vi "堆物理参数设置.vi"() -> ()   [LabVIEW 2020]
uses:
  global/SettingVariable.vi
  <vilib>/Utility/config.llb/Write Key (Double).vi
  GlobalVariable.vi
  TCPModbus_MasterClient/MB Ethernet Master Query Write Multiple Registers (poly).vi
  <vilib>/Utility/config.llb/NI_LVConfig.lvlib
panel:
  in  "下发":bool
  in  "Lamda 6":sgl caption="Lamda 6:"
  in  "Lamda 5":sgl caption="Lamda 5:"
  in  "Lamda 4":sgl caption="Lamda 4:"
  in  "Lamda 3":sgl caption="Lamda 3:"
  in  "Lamda 2":sgl caption="Lamda 2:"
  in  "βeff 6":sgl caption="βeff 6:"
  in  "βeff 5":sgl caption="βeff 5:"
  in  "βeff 4":sgl caption="βeff 4:"
  in  "βeff 3":sgl caption="βeff 3:"
  in  "βeff 2":sgl caption="βeff 2:"
  in  "取消":bool caption="Cancel Button"
  in  "确定":bool
  in  "Lamda 1":sgl caption="Lamda 1:"
  in  "βeff 1":sgl caption="βeff 1:"
  in  "源强":sgl caption="源强(n/cm2·s):"
  in  "中子寿命":sgl caption="中子寿命(s):"
  # "中子学参数"
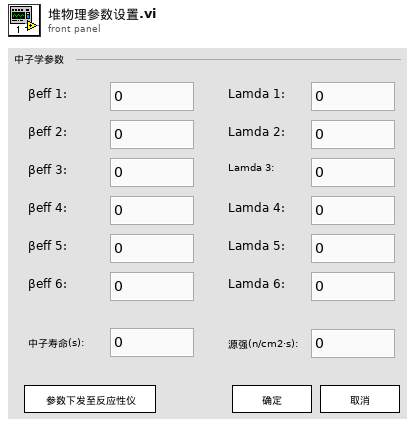
[diagram p1: front panel]
types:
  T1 = typedef "NI_LVConfig.lvlib/Config Data RefNum.ctl" = refnum<k1>
  T2 = enum32{"Bad", "Idle", "Run top level", "Running"}
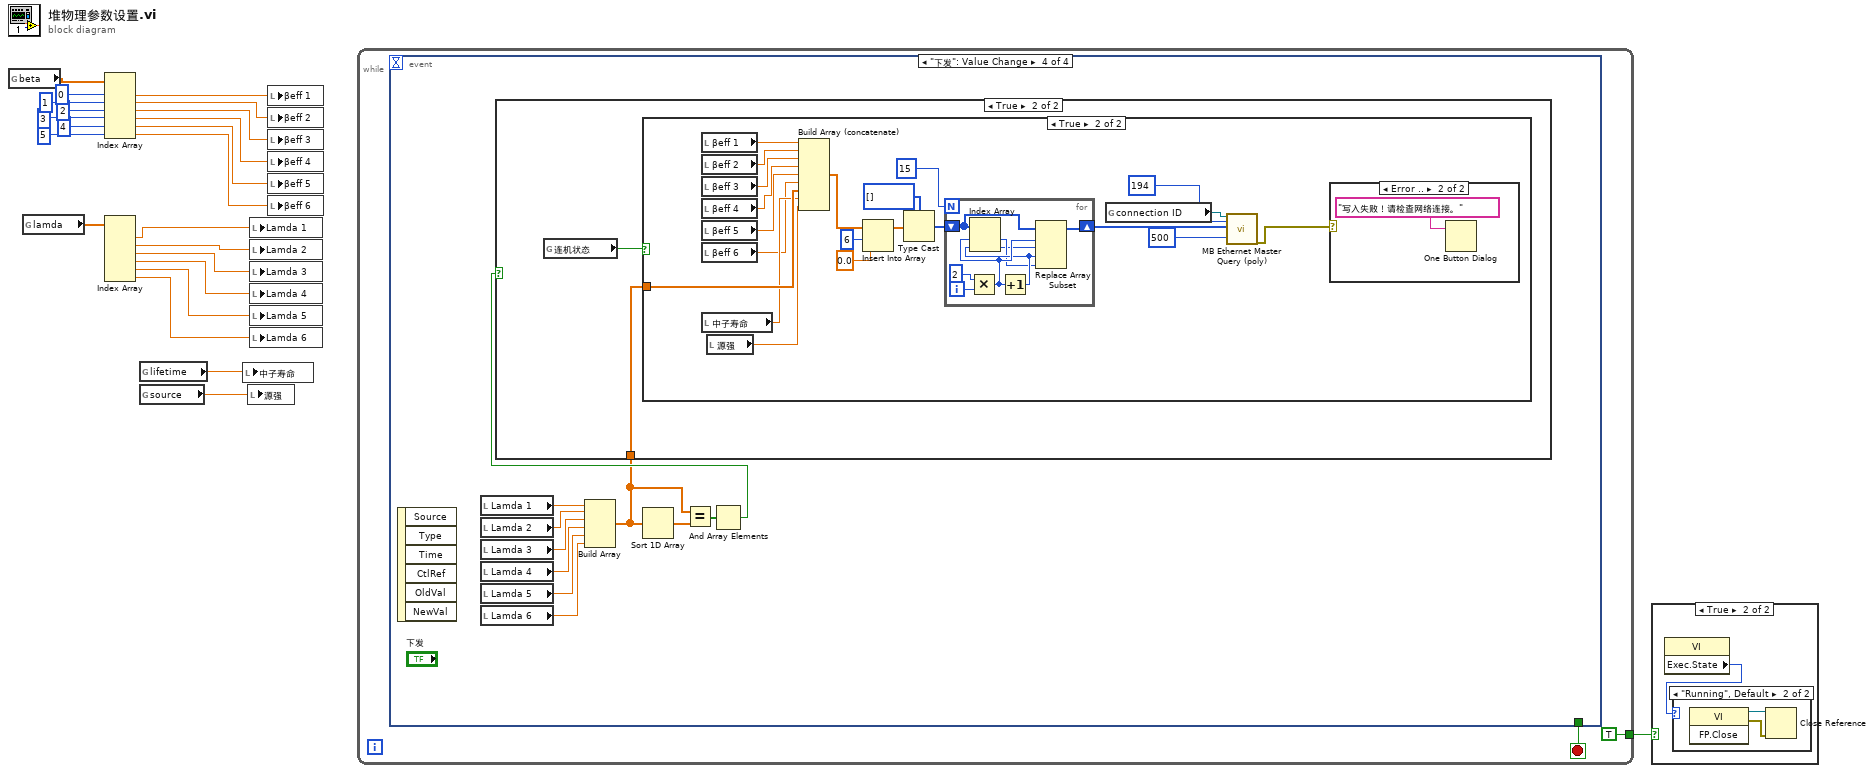
[diagram p0: block diagram]
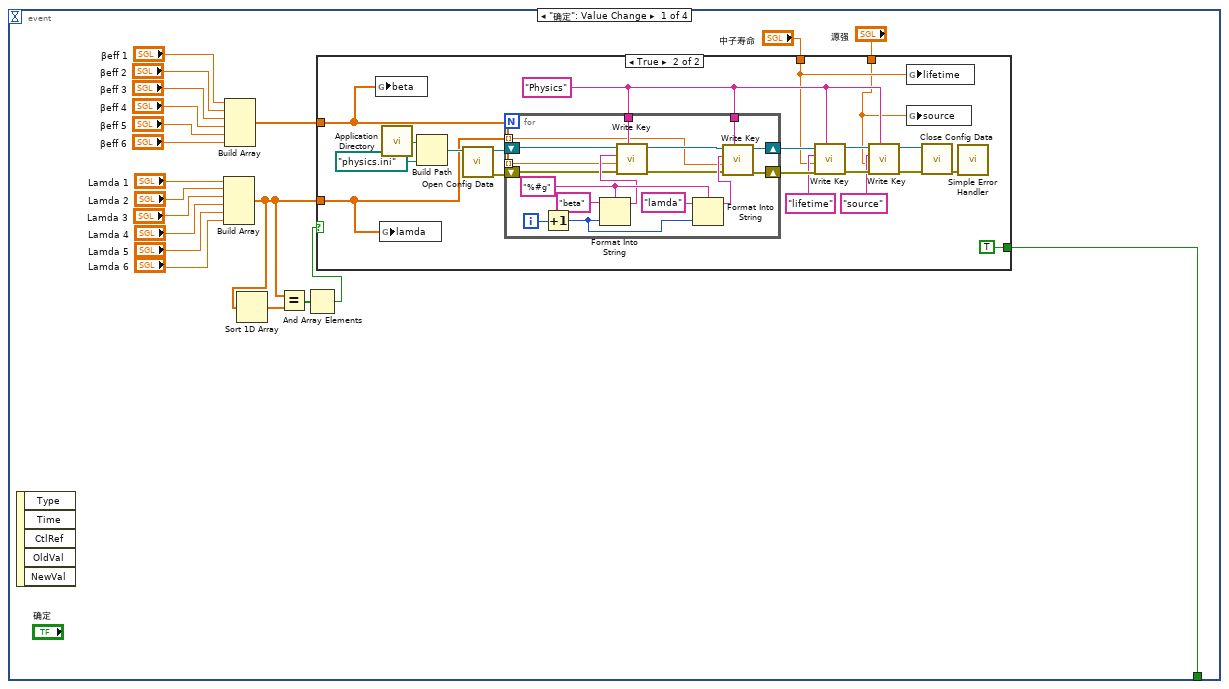
[diagram p4: hidden frame]
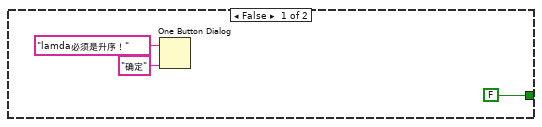
[diagram p5: hidden frame]
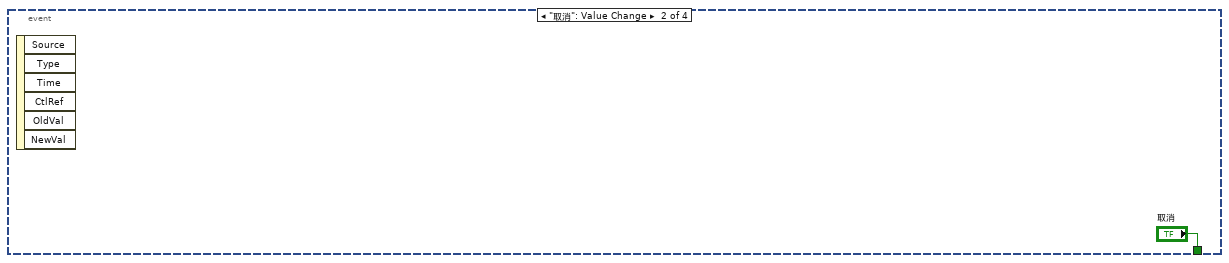
[diagram p6: hidden frame]
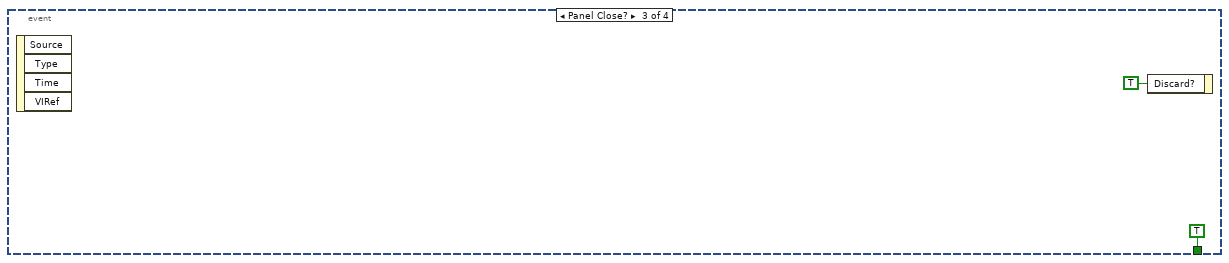
[diagram p7: hidden frame]
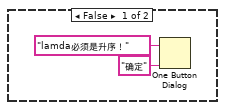
[diagram p8: hidden frame]
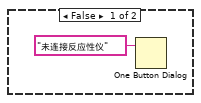
[diagram p9: hidden frame]
diagram:
  n1 = global read "SettingVariable.vi" "beta"() -> (w9:dbl[])
  n2 = global read "SettingVariable.vi" "lamda"() -> (w10:dbl[])
  n3 = Index Array(array=w9, index #1=0, index #2=1, index #3=2, index #4=3, index #5=4, index #6=5) -> (element #1=w17:dbl, element #2=w16:dbl, element #3=w15:dbl, element #4=w14:dbl, element #5=w13:dbl, element #6=w12:dbl)
  n4 = Index Array(array=w10) -> (element #1=w3:dbl, element #2=w4:dbl, element #3=w5:dbl, element #4=w6:dbl, element #5=w7:dbl, element #6=w8:dbl)  [unwired: 6 in]
  n5 = global read "SettingVariable.vi" "lifetime"() -> (w2:dbl)
  n6 = global read "SettingVariable.vi" "source"() -> (w1:dbl)
  n7 = local write "中子寿命"(w2) -> ()
  n8 = local write "源强"(w1) -> ()
  n9 = local write "Lamda 1"(w3) -> ()
  n10 = local write "Lamda 2"(w4) -> ()
  n11 = local write "Lamda 3"(w5) -> ()
  n12 = local write "Lamda 4"(w6) -> ()
  n13 = local write "Lamda 5"(w7) -> ()
  n14 = local write "Lamda 6"(w8) -> ()
  n15 = local write "βeff 1"(w17) -> ()
  n16 = local write "βeff 2"(w16) -> ()
  n17 = local write "βeff 3"(w15) -> ()
  n18 = local write "βeff 4"(w14) -> ()
  n19 = local write "βeff 5"(w13) -> ()
  n20 = local write "βeff 6"(w12) -> ()
  n21 = while {
    tunnel: [TRUE ("确定")] -> w11
    stop <- w25 stop-if-true
    n22 = event shown="[3] \"下发\": Value Change" {
      selector: _ -> [_ _ _ _]
      dyn-events: _ -> [_ _ _ _]
      timeout: _ -> [_ _ _ _]
      tunnel: [w26 "取消" TRUE ("确定") _] -> w25
      event "确定": Value Change {
        n23 = event-data() -> ()  [unwired: 1 in, 5 out]
        n24 = Build Array("Lamda 1", "Lamda 2", "Lamda 3", "Lamda 4", "Lamda 5", "Lamda 6") -> (w30:sgl[])
        n25 = Build Array("βeff 1", "βeff 2", "βeff 3", "βeff 4", "βeff 5", "βeff 6") -> (w33:sgl[])
        n26 = Sort 1D Array(array=w30) -> (sorted array=w29:sgl[])
        n27 = Equal?(x=w30, y=w29) -> (x = y?=w28:bool[])
        n28 = And Array Elements(Boolean array=w28) -> (logical AND=w27:bool)
        n29 = case shown="True" w27 {
          tunnel: w33 -> [_ w52]
          tunnel: w30 -> [_ w53]
          tunnel: "中子寿命" -> [_ w51]
          tunnel: "源强" -> [_ w50]
          tunnel: [FALSE ("确定") TRUE ("确定")] -> w26
          frame False {
            n30 = One Button Dialog(message="lamda必须是升序！", button name ("OK")="确定") -> ()  [unwired: 1 out]
          }
          frame True {
            w62 = "Physics" ("initial string")
            n31 = global write "SettingVariable.vi" "beta"(w52) -> ()
            n32 = global write "SettingVariable.vi" "lamda"(w53) -> ()
            n33 = call <vilib>:"Application Directory.vi"() -> ("Application Directory"=w67:path)
            n34 = Build Path(base path=w67, name or relative path=path "physics.ini") -> (appended path=w66:path)
            n35 = call <vilib>:"Open Config Data.vi"("configuration file path"=w66) -> ("error out"=w64:errorcluster, "refnum"=w65:T1)  [unwired: 2 in, 7 out]
            n36 = for {
              tunnel: w62 -> [w78]
              tunnel: w62 -> [w77]
              tunnel: w52 -> [w76] mode=indexing
              tunnel: w53 -> [w71] mode=indexing
              shift-right: [w69] -> w61
              shift-left: w65 -> [w75]
              shift-right: [w70] -> w59
              shift-left: w64 -> [w74]
              i -> [w85]
              w81 = "%#g" ("section")
              n37 = Increment(x=w85) -> (x+1=w82:i32)
              n38 = Format Into String(format string=w81, initial string="beta", w82) -> (resulting string=w80:string)  [unwired: 1 in, 1 out]
              n39 = call-poly <vilib>:"Write Key.vi"("section"=w78, "error in (no error)"=w74, "value"=w76, "key"=w80, "refnum"=w75) -> ("error out"=w73:errorcluster, "refnum out"=w72:T1)  [unwired: 4 in, 1 out]
              n40 = Format Into String(format string=w81, initial string="lamda", w82) -> (resulting string=w79:string)  [unwired: 1 in, 1 out]
              n41 = call-poly <vilib>:"Write Key.vi"("section"=w77, "error in (no error)"=w73, "value"=w71, "key"=w79, "refnum"=w72) -> ("error out"=w70:errorcluster, "refnum out"=w69:T1)  [unwired: 4 in, 1 out]
            }
            n42 = call-poly <vilib>:"Write Key.vi"("section"=w62, "error in (no error)"=w59, "value"=w51, "key"="lifetime", "refnum"=w61) -> ("error out"=w58:errorcluster, "refnum out"=w60:T1)  [unwired: 4 in, 1 out]
            n43 = call-poly <vilib>:"Write Key.vi"("section"=w62, "error in (no error)"=w58, "value"=w50, "key"="source", "refnum"=w60) -> ("error out"=w56:errorcluster, "refnum out"=w57:T1)  [unwired: 4 in, 1 out]
            n44 = global write "SettingVariable.vi" "lifetime"(w51) -> ()
            n45 = global write "SettingVariable.vi" "source"(w50) -> ()
            n46 = call <vilib>:"Close Config Data.vi"("error in (no error)"=w56, "refnum"=w57) -> ("error out"=w63:errorcluster)  [unwired: 1 in, 8 out]
            n47 = call <vilib>:"Simple Error Handler.vi"("error in (no error)"=w63) -> ()  [unwired: 1 in, 8 out]
          }
        }
      }
      event "取消": Value Change {
        n48 = event-data() -> ()  [unwired: 1 in, 6 out]
      }
      event Panel Close? {
        n49 = event-data() -> ()  [unwired: 1 in, 4 out]
        n50 = event-data("Discard?"=TRUE) -> ()  [unwired: 1 in, 1 out]
      }
      event "下发": Value Change {
        n51 = event-data() -> ()  [unwired: 1 in, 6 out]
        n52 = local read "Lamda 1"() -> (w98:sgl)
        n53 = local read "Lamda 2"() -> (w97:sgl)
        n54 = local read "Lamda 3"() -> (w96:sgl)
        n55 = local read "Lamda 4"() -> (w95:sgl)
        n56 = local read "Lamda 5"() -> (w94:sgl)
        n57 = local read "Lamda 6"() -> (w93:sgl)
        n58 = Build Array(w98, w97, w96, w95, w94, w93) -> (w89:sgl[])
        n59 = Sort 1D Array(array=w89) -> (sorted array=w92:sgl[])
        n60 = Equal?(x=w89, y=w92) -> (x = y?=w91:bool[])
        n61 = And Array Elements(Boolean array=w91) -> (logical AND=w90:bool)
        n62 = case shown="True" w90 {
          tunnel: w89 -> [_ w101]
          frame False {
            n63 = One Button Dialog(message="lamda必须是升序！", button name ("OK")="确定") -> ()  [unwired: 1 out]
          }
          frame True {
            n64 = global read "GlobalVariable.vi" "连机状态"() -> (w102:bool)
            n65 = case shown="True" w102 {
              tunnel: w101 -> [_ w122]
              frame False {
                n66 = One Button Dialog(message="未连接反应性仪") -> ()  [unwired: 1 in, 1 out]
              }
              frame True {
                n67 = local read "βeff 1"() -> (w124:sgl)
                n68 = local read "βeff 2"() -> (w123:sgl)
                n69 = local read "βeff 3"() -> (w119:sgl)
                n70 = local read "βeff 4"() -> (w118:sgl)
                n71 = local read "βeff 5"() -> (w117:sgl)
                n72 = local read "βeff 6"() -> (w116:sgl)
                n73 = local read "中子寿命"() -> (w121:sgl)
                n74 = local read "源强"() -> (w120:sgl)
                n75 = Build Array (concatenate)(w124, w123, w119, w118, w117, w116, w122, w121, w120) -> (w108:sgl[])
                n76 = Insert Into Array(array=w108, index=6 ("索引"), new element=sgl 0.0 ("新元素/子数组")) -> (w115:sgl[])
                n77 = Type Cast(type=u16[] [] ("Input Registers"), x=w115) -> (*(type *) &x=w114:u16[])
                n78 = for {
                  N: 15 -> [_]
                  shift-right: [w126] -> w109
                  shift-left: w114 -> [w131]
                  i -> [w133]
                  n79 = Multiply(x=2, y=w133) -> (x*y=w130:i32)
                  n80 = Increment(x=w130) -> (x+1=w129:i32)
                  n81 = Index Array(array=w131, index #1=w130, index #2=w129) -> (element #1=w128:u16, element #2=w127:u16)
                  n82 = Replace Array Subset(array=w131, new element #1=w127, index #1=w130, new element #2=w128, index #2=w129) -> (w126:u16[])
                }
                n83 = global read "GlobalVariable.vi" "connection ID"() -> (w106:refnum<k5>)
                n84 = call-poly "MB Ethernet Master Query (poly).vi"("TCP Connection Refnum in"=w106, "Starting Address"=u16 194, "Registers"=w109, "Timeout"=u32 500) -> ("error out"=w104:errorcluster)  [unwired: 2 in, 13 out]
                n85 = case shown="Error .." w104 {
                  frame No Error {
                  }
                  frame Error {
                    n86 = One Button Dialog(message="写入失败！请检查网络连接。") -> ()  [unwired: 1 in, 1 out]
                  }
                }
              }
            }
          }
        }
      }
    }
  }
  n87 = case shown="True" w11 {
    frame False {
    }
    frame True {
      n88 = property class="VI"() -> ("Exec.State"=w134:T2)  [unwired: 2 in, 2 out]
      n89 = case shown="\"Running\", Default" w134 {
        frame "Run top level" {
        }
        frame "Running", Default {
          n90 = invoke class="VI" method="FP.Close"() -> (reference out=w135:refnum<vi>, error out=w136:errorcluster)  [unwired: 3 in, 1 out]
          n91 = Close Reference(reference=w135, error in (no error)=w136) -> ()  [unwired: 1 out]
        }
      }
    }
  }
